vi "ZMQ subscriber example do not use.vi"() -> ()   [LabVIEW 2020]
uses:
  <vilib>/addons/zeromq/socket_type.ctl
  <vilib>/addons/zeromq/socket_options.ctl
  <vilib>/addons/zeromq/zeromq.lvlib
  <vilib>/addons/zeromq/zmq_context.lvclass
  <vilib>/addons/zeromq/zmq_socket.lvclass
panel:
  out "x+1":i32
  in  "Display all data":bool
  out "error out":errorcluster
  out "data":string
  out "time between acq":dbl
  in  "Stop":bool
  out "message":string[](array[string])
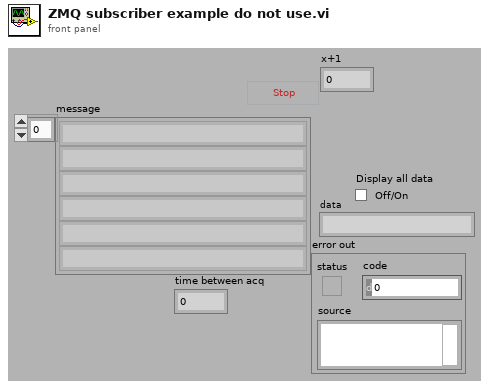
[diagram p1: front panel]
types:
  T1 = typedef "zeromq.lvlib/socket_options.ctl" = enum8{"NONE", "ZMQ_HWM", "<2>", "ZMQ_SWAP", "ZMQ_AFFINITY", "ZMQ_ROUTING_ID", "ZMQ_SUBSCRIBE", "ZMQ_UNSUBSCRIBE", "ZMQ_RATE", "ZMQ_RECOVERY_IVL", "ZMQ_MCAST_LOOP", "ZMQ_SNDBUF", "ZMQ_RCVBUF", "ZMQ_RCVMORE", "ZMQ_FD", "ZMQ_EVENTS", "ZMQ_TYPE", "ZMQ_LINGER", "ZMQ_RECONNECT_IVL", "ZMQ_BACKLOG", "ZMQ_RECOVERY_IVL_MSEC", "ZMQ_RECONNECT_IVL_MAX", "ZMQ_MAXMSGSIZE", "ZMQ_SNDHWM", "ZMQ_RCVHWM", "ZMQ_MULTICAST_HOPS", "<26>", "ZMQ_RCVTIMEO", "ZMQ_SNDTIMEO", "<29>", "<30>", "ZMQ_IPV4ONLY", "ZMQ_LAST_ENDPOINT", "ZMQ_ROUTER_MANDATORY", "ZMQ_TCP_KEEPALIVE", "ZMQ_TCP_KEEPALIVE_CNT", "ZMQ_TCP_KEEPALIVE_IDLE", "ZMQ_TCP_KEEPALIVE_INTVL", "ZMQ_TCP_ACCEPT_FILTER", "ZMQ_IMMEDIATE", "ZMQ_XPUB_VERBOSE", "ZMQ_ROUTER_RAW", "ZMQ_IPV6", "ZMQ_MECHANISM", "ZMQ_PLAIN_SERVER", "ZMQ_PLAIN_USERNAME", "ZMQ_PLAIN_PASSWORD", "ZMQ_CURVE_SERVER", "ZMQ_CURVE_PUBLICKEY", "ZMQ_CURVE_SECRETKEY", "ZMQ_CURVE_SERVERKEY", "ZMQ_PROBE_ROUTER", "ZMQ_REQ_CORRELATE", "ZMQ_REQ_RELAXED", "ZMQ_CONFLATE", "ZMQ_ZAP_DOMAIN", "ZMQ_ROUTER_HANDOVER", "ZMQ_TOS", "ZMQ_IPC_FILTER_PID", "ZMQ_IPC_FILTER_UID", "ZMQ_IPC_FILTER_GID", "ZMQ_CONNECT_ROUTING_ID", "ZMQ_GSSAPI_SERVER", "ZMQ_GSSAPI_PRINCIPAL", "ZMQ_GSSAPI_SERVICE_PRINCIPAL", "ZMQ_GSSAPI_PLAINTEXT", "ZMQ_HANDSHAKE_IVL", "<67>", "ZMQ_SOCKS_PROXY", "ZMQ_XPUB_NODROP", "ZMQ_BLOCKY", "ZMQ_XPUB_MANUAL", "ZMQ_XPUB_WELCOME_MSG", "ZMQ_STREAM_NOTIFY", "ZMQ_INVERT_MATCHING", "ZMQ_HEARTBEAT_IVL", "ZMQ_HEARTBEAT_TTL", "ZMQ_HEARTBEAT_TIMEOUT", "ZMQ_XPUB_VERBOSER", "ZMQ_CONNECT_TIMEOUT", "ZMQ_TCP_MAXRT", "ZMQ_THREAD_SAFE", "<82>", "<83>", "ZMQ_MULTICAST_MAXTPDU", "ZMQ_VMCI_BUFFER_SIZE", "ZMQ_VMCI_BUFFER_MIN_SIZE", "ZMQ_VMCI_BUFFER_MAX_SIZE", "ZMQ_VMCI_CONNECT_TIMEOUT", "ZMQ_USE_FD", "ZMQ_GSSAPI_PRINCIPAL_NAMETYPE", "ZMQ_GSSAPI_SERVICE_PRINCIPAL_NAMETYPE", "ZMQ_BINDTODEVICE", "ZMQ_ZAP_ENFORCE_DOMAIN", "ZMQ_LOOPBACK_FASTPATH", "ZMQ_METADATA", "ZMQ_MULTICAST_LOOP", "ZMQ_ROUTER_NOTIFY"}
  T2 = typedef "zeromq.lvlib/socket_type.ctl" = enum8{"ZMQ_PAIR", "ZMQ_PUB", "ZMQ_SUB", "ZMQ_REQ", "ZMQ_REP", "ZMQ_DEALER", "ZMQ_ROUTER", "ZMQ_PULL", "ZMQ_PUSH", "ZMQ_XPUB", "ZMQ_XSUB", "ZMQ_STREAM", "ZMQ_SERVER", "ZMQ_CLIENT", "ZMQ_RADIO", "ZMQ_DISH", "ZMQ_GATHER", "ZMQ_SCATTER", "ZMQ_DGRAM"}
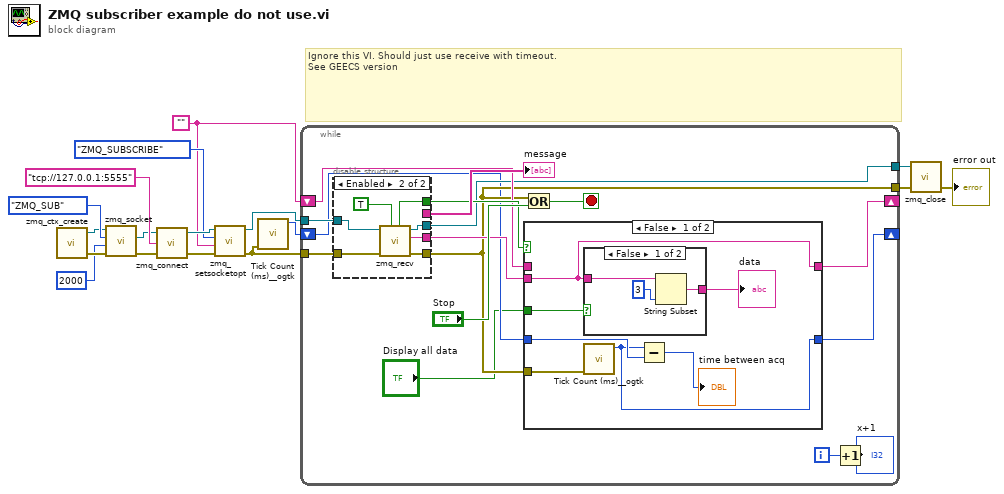
[diagram p0: block diagram]
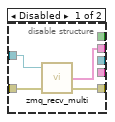
[diagram p4: hidden frame]
diagram:
  w4 = ""
  # "Ignore this VI. Should just use receive with timeout.\nSee GEECS version"
  n1 = call <vilib>:"zmq_ctx_create.vi"() -> ("error out"=w16:errorcluster, "context out"=w8:refnum<class "zmq_context.lvclass">)  [unwired: 4 in]
  n2 = call <vilib>:"zmq_socket.vi"("error in"=w16, "linger (ms)"=2000, "socket type"=socket_type."ZMQ_SUB", "context in"=w8) -> ("error out"=w15:errorcluster, "socket out"=w9:refnum<class "zmq_socket.lvclass">)  [unwired: 1 in, 1 out]
  n3 = call <vilib>:"zmq_connect.vi"("error in"=w15, "endpoint"="tcp://127.0.0.1:5555", "socket in"=w9) -> ("error out"=w13:errorcluster, "socket out"=w14:refnum<class "zmq_socket.lvclass">)  [unwired: 1 in]
  n4 = call <vilib>:"zmq_setsocketopt.vi"("error in"=w13, "value"=w4, "option"=socket_options."ZMQ_SUBSCRIBE", "socket in"=w14) -> ("error out"=w7:errorcluster, "socket out"=w12:refnum<class "zmq_socket.lvclass">)  [unwired: 2 in]
  n5 = call <userlib>:"Tick Count (ms)__ogtk.vi"("error in (no error)"=w7) -> ("millisecond timer value"=w6:u32)  [unwired: 9 in, 1 out]
  n6 = while {
    tunnel: w12 -> [w33]
    tunnel: w7 -> [w31]
    tunnel: [w22] -> w3
    shift-right: [w26] -> _
    shift-left: w4 -> [w24]
    tunnel: [w23] -> w2
    shift-right: [w20] -> _
    shift-left: w6 -> [w21]
    i -> [w28]
    stop <- w29 stop-if-true
    n7 = disable-structure shown="Enabled" {
      disable-tunnel: w33 -> [w50 w57]
      disable-tunnel: [w49 _] -> w32
      disable-tunnel: w31 -> [w48 w56]
      disable-tunnel: [w47 w55] -> w22
      disable-tunnel: [_ w53] -> w27
      disable-tunnel: [_ w52] -> w25
      disable-tunnel: [_ w51] -> w23
      frame Disabled {
        n8 = call <vilib>:"zmq_recv_multi.vi"("error in"=w48, "socket in"=w50) -> ("error out"=w47:errorcluster, "parts"=w49:string[])  [unwired: 1 in, 1 out]
      }
      frame Enabled {
        n9 = call <vilib>:"zmq_recv.vi"("no block? (F)"=TRUE, "error in"=w56, "socket in"=w57) -> ("error out"=w55:errorcluster, "data"=w52:string, "socket out"=w51:refnum<class "zmq_socket.lvclass">, "timeout?"=w53:bool)  [unwired: 2 in, 1 out]
      }
    }
    "message" <- w32
    n10 = Or(x=w22, y="Stop") -> (x .or. y?=w29:bool)
    n11 = case shown="False" w27 {
      tunnel: [w35 w46] -> w26
      tunnel: w25 -> [w35 _]
      tunnel: w24 -> [_ w46]
      tunnel: w22 -> [w40 _]
      tunnel: w21 -> [w39 w45]
      tunnel: [w37 w45] -> w20
      tunnel: "Display all data" -> [w34 _]
      frame False {
        n12 = case shown="False" w34 {
          tunnel: [w43 w44] -> w36
          tunnel: w35 -> [w42 w44]
          frame False {
            n13 = String Subset(string=w42, length (rest)=3 ("length (rest)")) -> (substring=w43:string)  [unwired: 1 in]
          }
          frame True {
          }
        }
        "data" <- w36
        n14 = call <userlib>:"Tick Count (ms)__ogtk.vi"("error in (no error)"=w40) -> ("millisecond timer value"=w37:u32)  [unwired: 9 in, 1 out]
        n15 = Subtract(x=w37, y=w39) -> (x-y=→"time between acq":u32)
      }
      frame True {
      }
    }
    n16 = Increment(x=w28) -> (x+1=→"x+1":i32)
  }
  n17 = call <vilib>:"zmq_close.vi"("error in"=w3, "socket"=w2) -> ("error out"=→"error out":errorcluster)  [unwired: 3 in]
